vi "AM_1019.vi"() -> ()   [LabVIEW 2019]
uses:
  <vilib>/express/express analysis/Spectral/Block/exnSpectralBlock spectral measurements RMS poly.vi
  <vilib>/express/express analysis/Spectral/XNode/ExpressSpectralMeasurementsBlockNode.xnode
  <vilib>/express/express analysis/Spectral/Block/exnSpectralBlock spectral measurements RMS DDT.vi
panel:
  in  "AM":dbl
  in  "DC":dbl
  in  "stop":bool
  in  "Message Freq(HZ)":dbl(slide) scale=0.0..1000.0
  in  "Carrier Freq(HZ)":dbl(slide) scale=0.0..10000.0
  out "Spectrum":dynamicdata(graph)
  out "Message Signal":dynamicdata(graph)
  out "Modulated Signal":dynamicdata(graph)
  out "Carrier Signal":dynamicdata(graph)
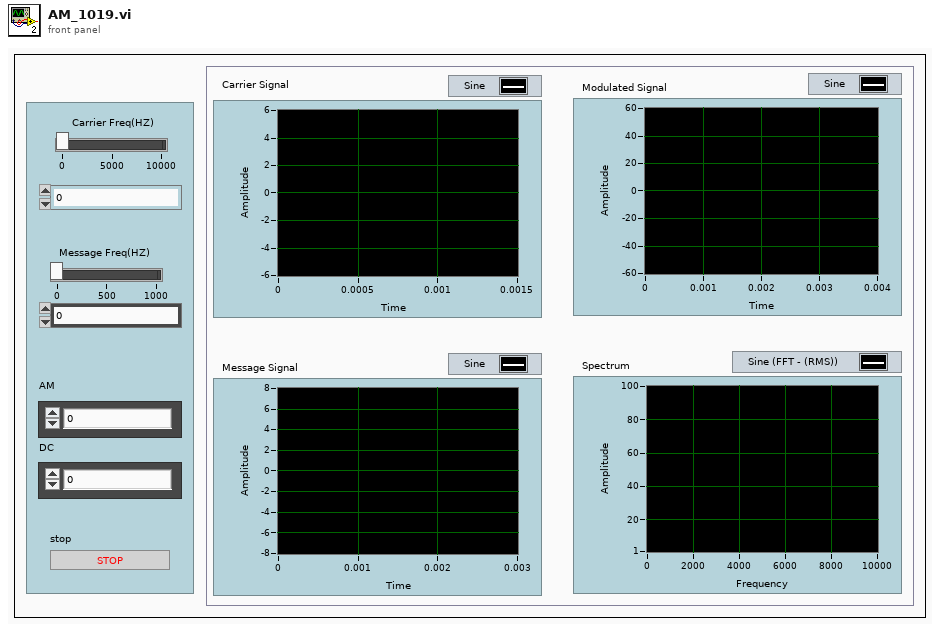
[diagram p1: front panel]
types:
  T1 = cluster{"averaging mode":u16, "weighting mode":u16, "number of averages":u32}
  T2 = cluster{"dB On (F)":bool, "unwrap phase (F)":bool, "convert to degree (F)":bool}
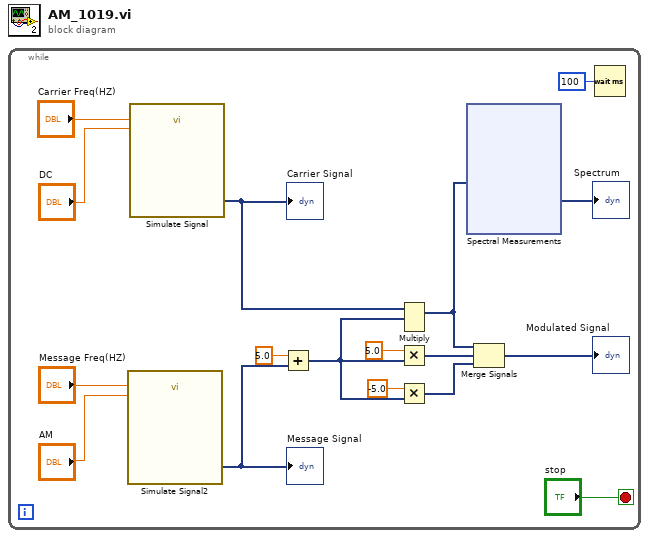
[diagram p0: block diagram]
diagram:
  n1 = while {
    stop <- "stop" stop-if-true
    n2 = call "Simulate Signal2"("Frequency"="Message Freq(HZ)", "Amplitude"="AM") -> ("Sine"=w13:dynamicdata)  [unwired: 12 in, 1 out]
    "Message Signal" <- w13
    n3 = call "Simulate Signal"("Frequency"="Carrier Freq(HZ)", "Amplitude"="DC") -> ("Sine"=w17:dynamicdata)  [unwired: 12 in, 1 out]
    "Carrier Signal" <- w17
    n4 = Add(x=5.0, y=w13) -> (x+y=w12:dynamicdata)
    n5 = Multiply(1:w12, 2:w17) -> (0:w4:dynamicdata)  [unwired: 1 in, 1 out]
    n6 = Multiply(x=5.0, y=w12) -> (x*y=w10:dynamicdata)
    n7 = Multiply(x=-5.0, y=w12) -> (x*y=w11:dynamicdata)
    n8 = xnode "Spectral Measurements"("Signals"=w4) -> ("FFT - (RMS)"=→"Spectrum":dynamicdata)  [unwired: 1 in, 2 out]
    n9 = Merge Signals(w4, w10, w11) -> (→"Modulated Signal":dynamicdata)
    n10 = Wait (ms)(milliseconds to wait=u32 100) -> ()  [unwired: 1 out]
  }
